vi "APTpiezoGet.vi"(8 "error in (no error)":errorcluster, 11 "reference":refnum<k7>) -> (0 "error out":errorcluster, 2 "pfPosition":sgl, 3 "reference out":refnum<k7>)   [LabVIEW 2016]
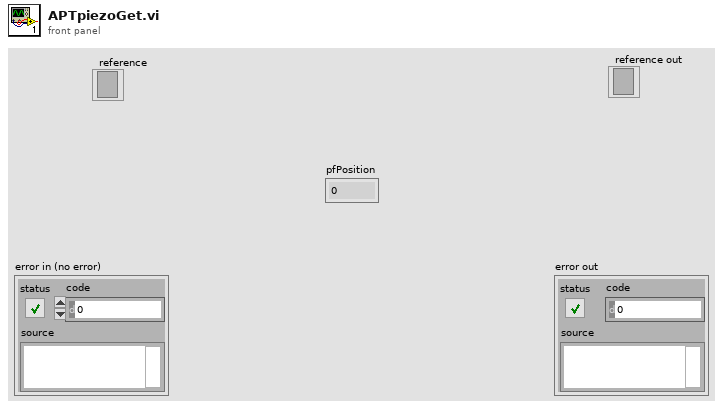
[diagram p1: front panel]
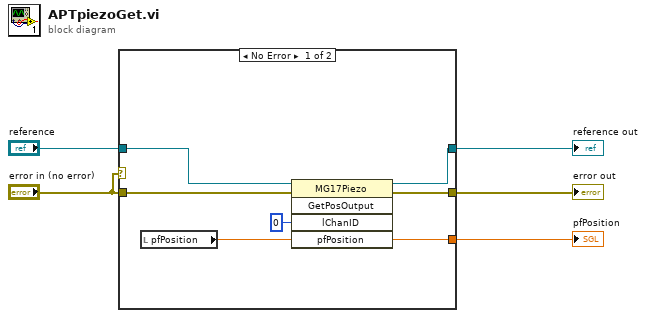
[diagram p0: block diagram]
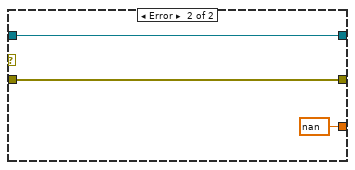
[diagram p2: hidden frame]
diagram:
  n1 = case shown="No Error" "error in (no error)" {
    tunnel: [w12 w15] -> w5
    tunnel: "error in (no error)" -> [w10 w14]
    tunnel: [w9 w14] -> w4
    tunnel: "reference" -> [w8 w15]
    tunnel: [w7 sgl nan ("pfPosition")] -> w2
    frame No Error {
      n2 = local read "pfPosition"() -> (w6:sgl)
      n3 = invoke class="MG17Piezo" method="GetPosOutput"(reference=w8, error in=w10, "lChanID"=0, "pfPosition"=w6) -> (reference out=w12:refnum<k7>, error out=w9:errorcluster, "pfPosition"=w7:sgl)  [unwired: 1 in, 2 out]
    }
    frame Error {
    }
  }
  "error out" <- w4
  "reference out" <- w5
  "pfPosition" <- w2
